vi "基本运动参考例程 - Copy.vi"() -> ()   [LabVIEW 2020]
uses:
  VIs/gts.lvlib
panel:
  in  "pPrm 3":cluster{"acc":dbl, "dec":dbl, "smooth":dbl}={"acc"=1.0, "dec"=1.0, "smooth"=0.0}
  in  "vel 2":dbl=30.0
  in  "Jog运动":bool
  in  "pos":i32=20000
  in  "vel":dbl=30.0
  in  "pPrm":T1={"acc"=1.0, "dec"=1.0, "velStart"=0.0, "smoothTime"=20}
  in  "点位运动":bool
  in  "数据路径":path
  in  "pCrdPrm":T2={"dimension"=2, "profile[0]"=1, "profile[1]"=2, "profile[2]"=0, "profile[3]"=0, "profile[4]"=0, "profile[5]"=0, "profile[6]"=0, "profile[7]"=0, "@dummy control@"=0, "@dummy control@"=0, "@dummy control@"=0, "@dummy control@"=0, "@dummy control@"=0, "@dummy control@"=0, "synVelMax"=500.0, "synAccMax"=1.0, "evenTime"=10, "setOriginFlag"=0, "originPos[0]"=0, "originPos[1]"=0, "originPos[2]"=0, "originPos[3]"=0, "originPos[4]"=0, "originPos[5]"=0, "originPos[6]"=0, "originPos[7]"=0}
  in  "前瞻":bool
  in  "插补运动":bool
  in  "pLookAheadBuf":T3(array[cluster])
  out "pStatus out":i16
  in  "轴号":T4(ring)=enum."1"
  in  "一维线性输出":bool
  in  "类型":u16(ring) items=["脉冲", "电平"]
  in  "单次输出":bool
  out "闭环返回值":i16[](array[numeric])
  in  "闭环PID参数":T5={"kp"=2.0, "ki"=0.0, "kd"=0.0, "kvff"=0.0, "kaff"=0.0, "integralLimit"=0, "derivativeLimit"=0, "limit"=32767}
  in  "闭环控制":bool
  out "updatemotion return":i16
  in  "更新运动":bool
  out "0号模块DI0输入":u16
  out "ExIoLoad return":i16
  out "openEXIO return":i16
  in  "扩展IO模块":bool
  out "2Dclear return":i16
  out "zero return":i16
  in  "清零":bool
  out "CrdStart return":i16
  out "二维输出次数":i32
  out "一维输出次数":i32[](array[numeric])
  out "1Dstatus return":i16
  in  "查询位置比较状态":bool
  out "2Dsetpara return":i16
  in  "二维位置比较参数设置":T6={"encx"=1, "ency"=2, "source"=1, "outputType"=0, "startLevel"=0, "time"=30, "maxerr"=100, "threshold"=0}
  out "se2Dcompare return":i16
  out "2Ddata return":i16
  in  "二维位置数组":cluster{"px":i32, "py":i32}[](array[cluster])=[{"px"=10000, "py"=10000}, {"px"=20000, "py"=20000}, {"px"=30000, "py"=30000}]
  out "1Dcompare return":i16
  in  "一维位置数组":dbl[](array[numeric])=[10000.0, 20000.0, 30000.0]
  out "crddata return":i16
  out "Lnxy return":i16
  out "setCrd return":i16
  out "lookahead":i16
  in  "二维位置比较":bool
  in  "一维位置比较":bool
  out "实际速度":dbl[](array[numeric])
  out "getenc return":i16
  out "实际位置":dbl[](array[numeric])
  out "encvel return":i16
  out "规划位置":dbl[](array[numeric])
  out "prfpos return":i16
  out "规划速度":dbl[](array[numeric])
  out "prfvel return":i16
  out "homezero return":i16
  out "gethomests return":i16
  out "pHomeStatus out":T7
  out "gohome return":i16
  out "get home prm return":i16
  in  "pHomePrm":T8={"mode"=20, "moveDir"=1, "indexDir"=1, "edge"=0, "triggerIndex"=-1, "pad1[0]"=0, "pad1[1]"=0, "pad1[2]"=0, "velHigh"=10.0, "velLow"=3.0, "acc"=0.1, "dec"=0.1, "smoothTime"=20, "pad2[0]"=0, "pad2[1]"=0, "pad2[2]"=0, "homeOffset"=1000, "searchHomeDistance"=0, "searchIndexDistance"=0, "escapeStep"=0, "pad3[0]"=0, "pad3[1]"=0}
  out "JogStop return":i16
  out "Update return":i16
  out "setVel return":i16
  out "setPrm return":i16
  out "getPrm return":i16
  out "PrfJog return":i16
  in  "回原点":bool
  out "reset return":i16
  out "Axisoff return":i16
  out "stopreturn":i16
  out "updatereturn":i16
  out "pos return":i16
  out "vel return":i16
  out "set prmreturn":i16
  out "get prm return":i16
  out "set trap return":i16
  out "Axison return":i16
  out "clrsts return":i16
  out "config return":i16
  in  "路径":path=path "D:/王淼清/控制卡常用功能例程(Labview)/GTS800.cfg"
  out "open return":i16
  in  "关伺服":bool
  in  "停止":bool
  in  "开伺服":bool
  in  "开卡":bool
  # "查询位置比较状态"
  # "插补运动参数"
  # "操作步骤：\n①按开卡键，打开卡和复位；\n②按开伺服键，1轴使能；\n③按点位键，1轴运动；\n注意事项：\n①按键时，时间不能太短，稍微长按一会；\n③在按键前，先设置各参数；\n④需要停止时，按停止键。\n参数说明：\naxis：运动轴，范围为1-8；\nvel：当前轴的轴速；\npos：当前轴的规划位置；\npPrm：点位运动的参数设置，可参考编程手册；\nconfig：配置文件，具体参数设置参考编程手册；\n备注：\n本例程函数返回值都以显示控件表示，函数名称在\n显示控件上方，每个函数都对应有一个显示控件，\n重复调用函数，只对应一个显示控件；"
  # "位置速度显示"
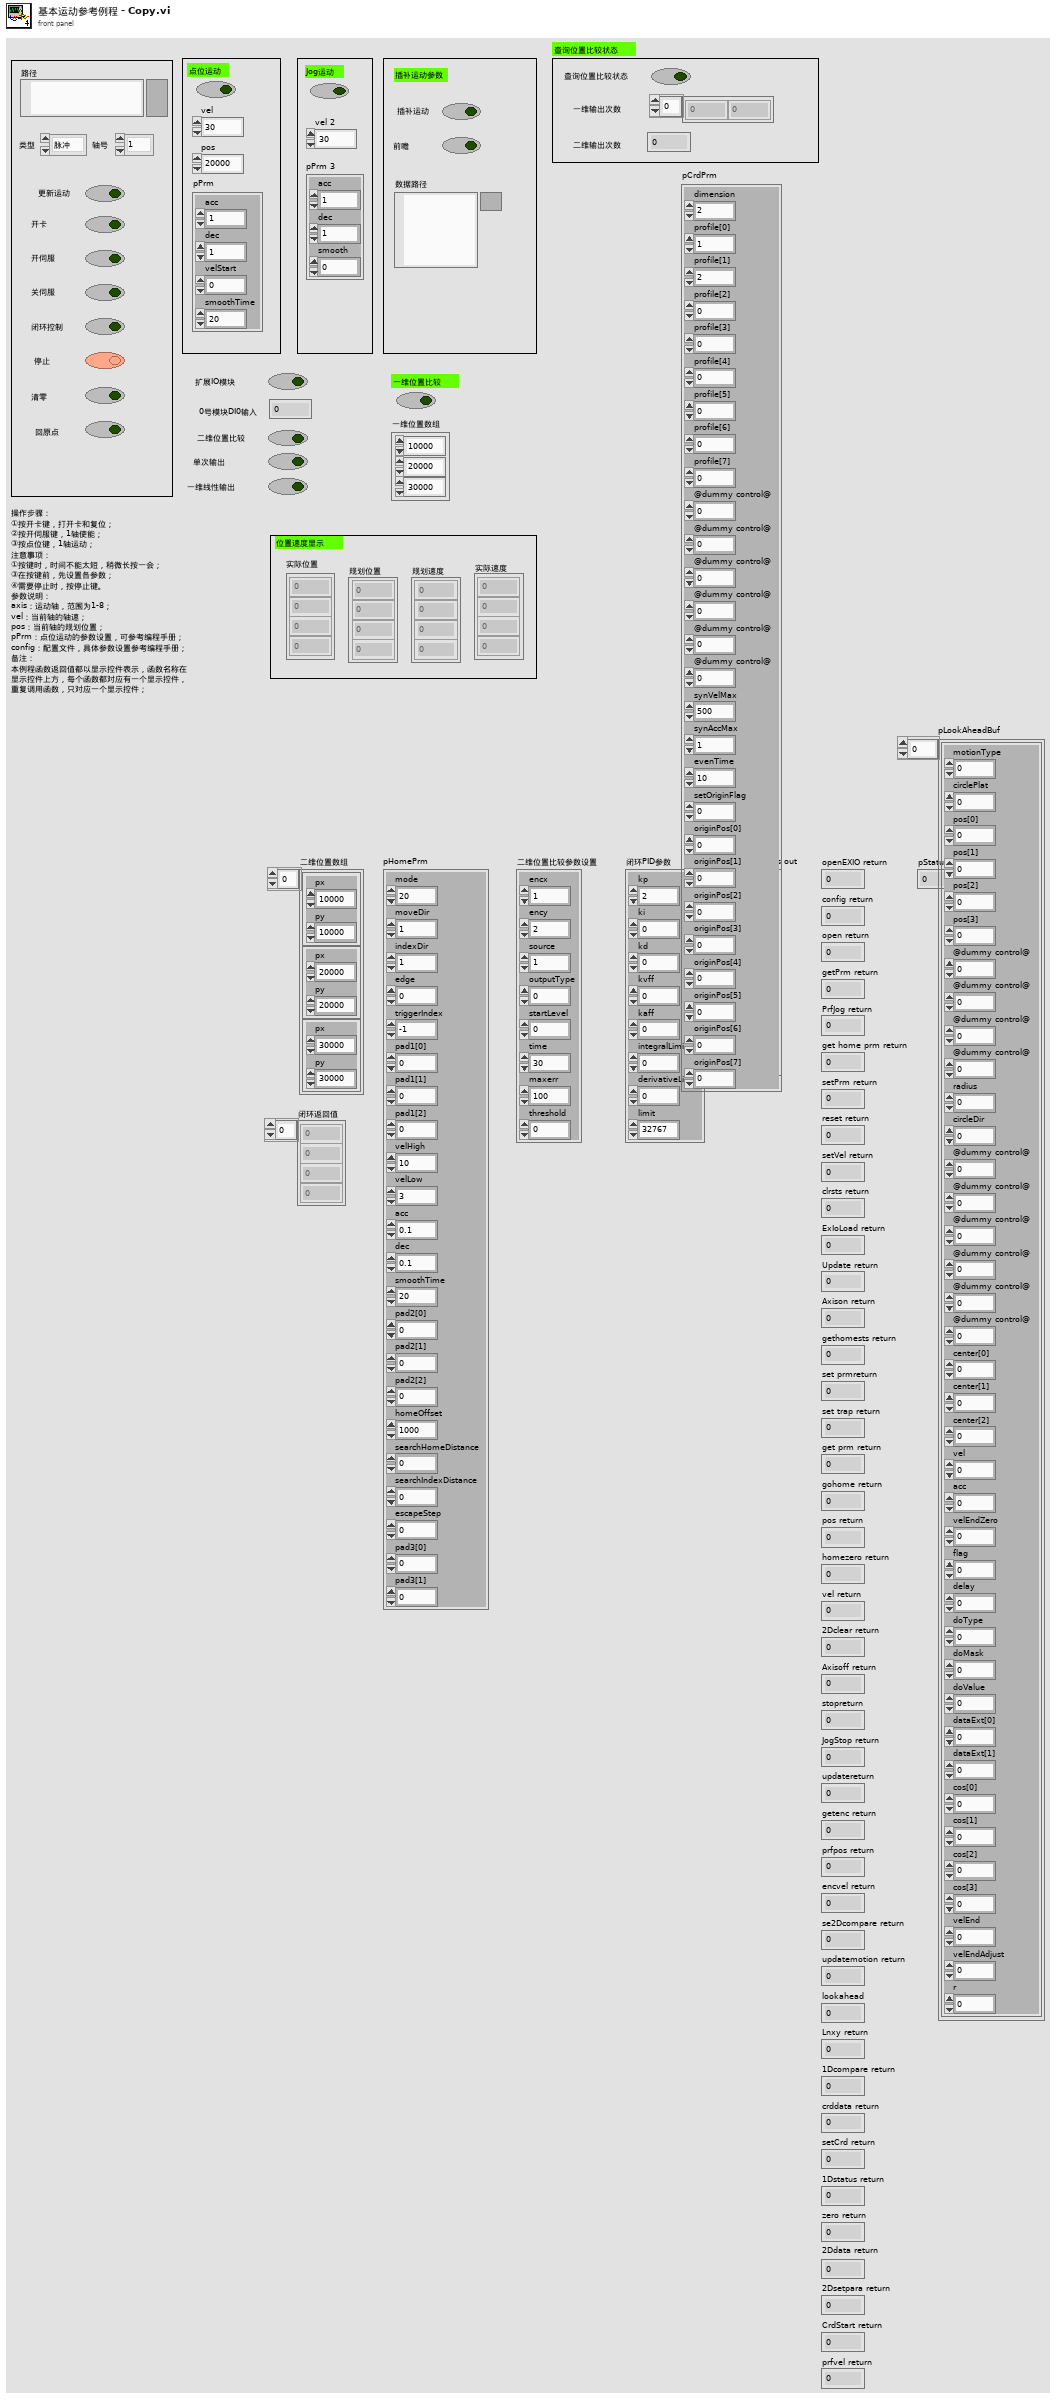
[diagram p1: front panel]
types:
  T1 = cluster{"acc":dbl, "dec":dbl, "velStart":dbl, "smoothTime":i16}
  T2 = cluster{"dimension":i16, "profile[0]":i16, "profile[1]":i16, "profile[2]":i16, "profile[3]":i16, "profile[4]":i16, "profile[5]":i16, "profile[6]":i16, "profile[7]":i16, "@dummy control@":i8, "@dummy control@":i8, "@dummy control@":i8, "@dummy control@":i8, "@dummy control@":i8, "@dummy control@":i8, "synVelMax":dbl, "synAccMax":dbl, "evenTime":i16, "setOriginFlag":i16, "originPos[0]":i32, "originPos[1]":i32, "originPos[2]":i32, "originPos[3]":i32, "originPos[4]":i32, "originPos[5]":i32, "originPos[6]":i32, "originPos[7]":i32}
  T3 = cluster{"motionType":i16, "circlePlat":i16, "pos[0]":i32, "pos[1]":i32, "pos[2]":i32, "pos[3]":i32, "@dummy control@":i8, "@dummy control@":i8, "@dummy control@":i8, "@dummy control@":i8, "radius":dbl, "circleDir":i16, "@dummy control@":i8, "@dummy control@":i8, "@dummy control@":i8, "@dummy control@":i8, "@dummy control@":i8, "@dummy control@":i8, "center[0]":dbl, "center[1]":dbl, "center[2]":dbl, "vel":dbl, "acc":dbl, "velEndZero":i16, "flag":i16, "delay":u16, "doType":i16, "doMask":u16, "doValue":u16, "dataExt[0]":u16, "dataExt[1]":u16, "cos[0]":dbl, "cos[1]":dbl, "cos[2]":dbl, "cos[3]":dbl, "velEnd":dbl, "velEndAdjust":dbl, "r":dbl}[]
  T4 = enum16{"none", "1", "2", "3", "4", "5", "6", "7", "8"}
  T5 = cluster{"kp":dbl, "ki":dbl, "kd":dbl, "kvff":dbl, "kaff":dbl, "integralLimit":i32, "derivativeLimit":i32, "limit":i16}
  T6 = cluster{"encx":i16, "ency":i16, "source":i16, "outputType":i16, "startLevel":i16, "time":i16, "maxerr":i16, "threshold":i16}
  T7 = cluster{"run":i16, "stage":i16, "error":i16, "pad1":i16, "capturePos":i32, "targetPos":i32}
  T8 = cluster{"mode":i16, "moveDir":i16, "indexDir":i16, "edge":i16, "triggerIndex":i16, "pad1[0]":i16, "pad1[1]":i16, "pad1[2]":i16, "velHigh":dbl, "velLow":dbl, "acc":dbl, "dec":dbl, "smoothTime":i16, "pad2[0]":i16, "pad2[1]":i16, "pad2[2]":i16, "homeOffset":i32, "searchHomeDistance":i32, "searchIndexDistance":i32, "escapeStep":i32, "pad3[0]":i32, "pad3[1]":i32}
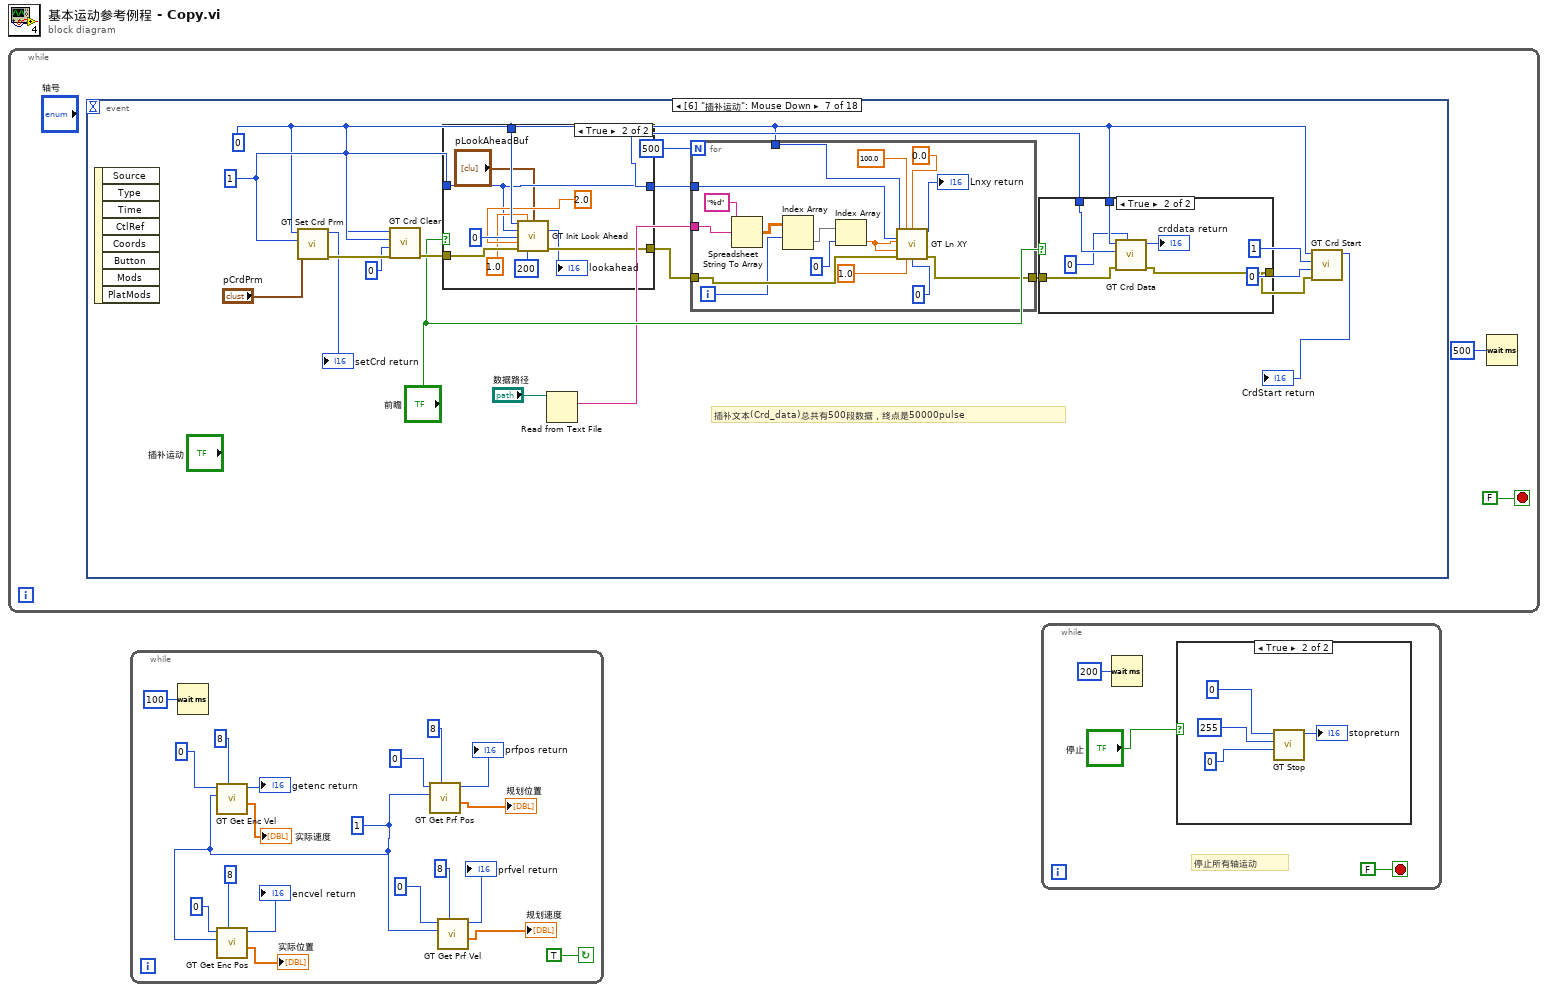
[diagram p0: block diagram]
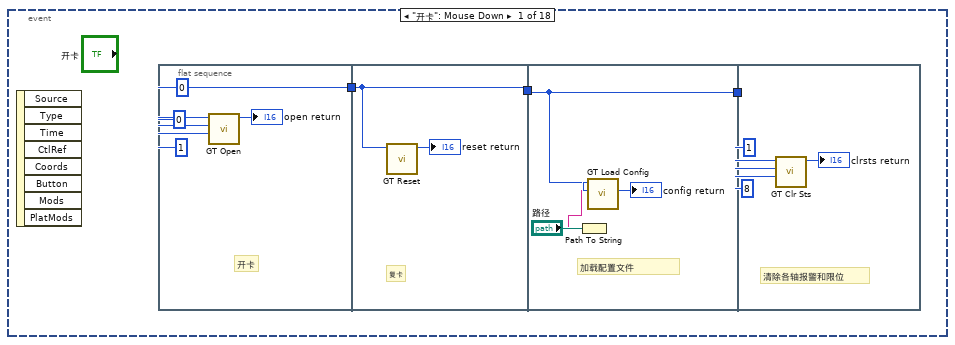
[diagram p3: hidden frame]
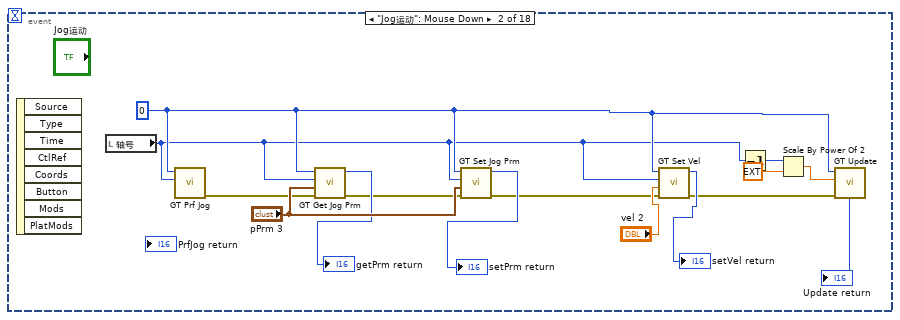
[diagram p4: hidden frame]
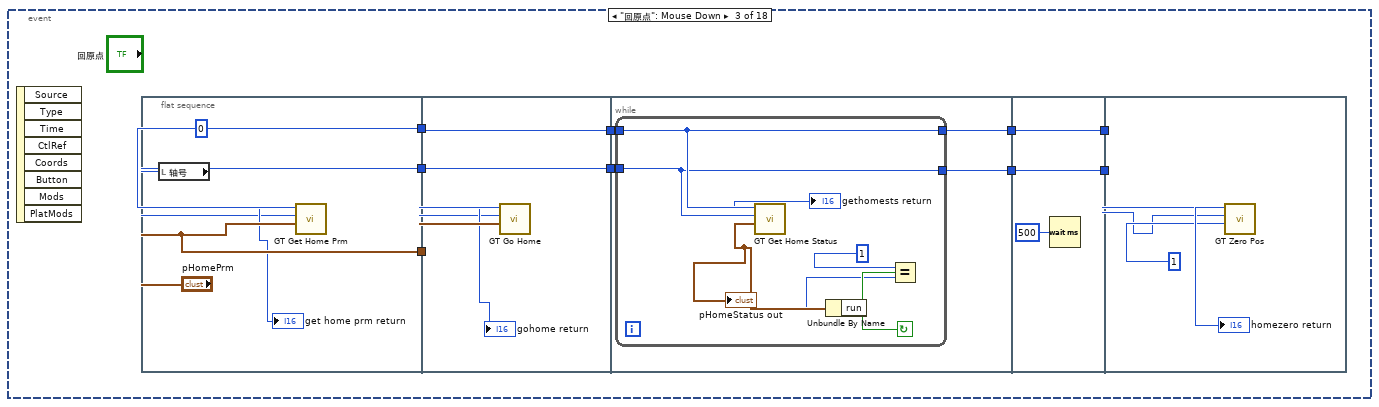
[diagram p5: hidden frame]
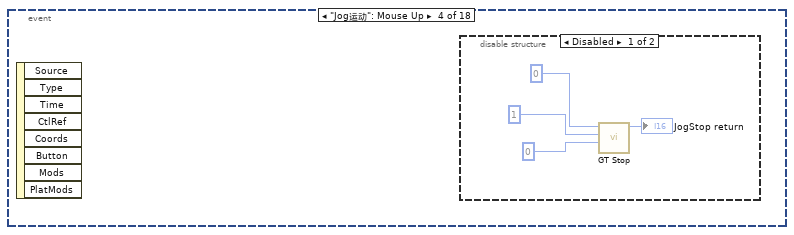
[diagram p6: hidden frame]
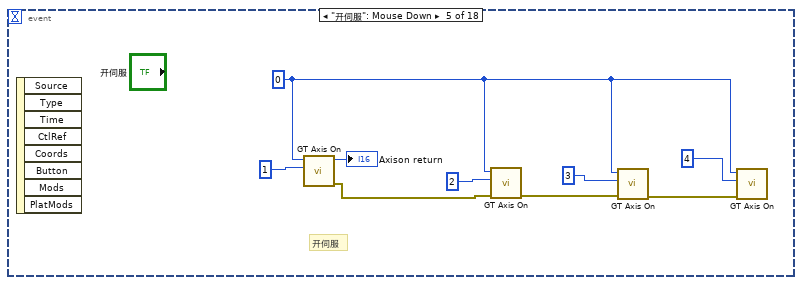
[diagram p8: hidden frame]
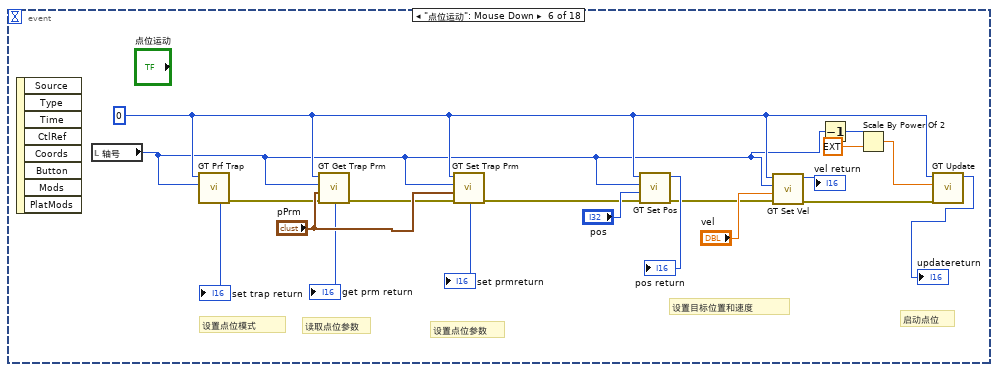
[diagram p9: hidden frame]
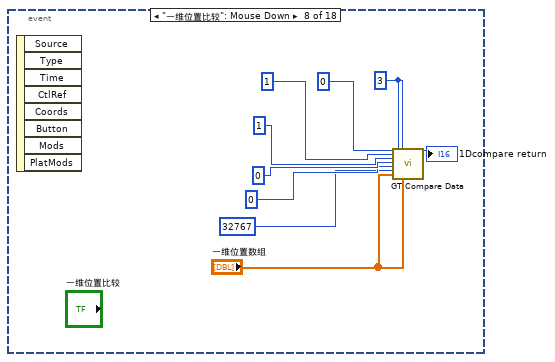
[diagram p12: hidden frame]
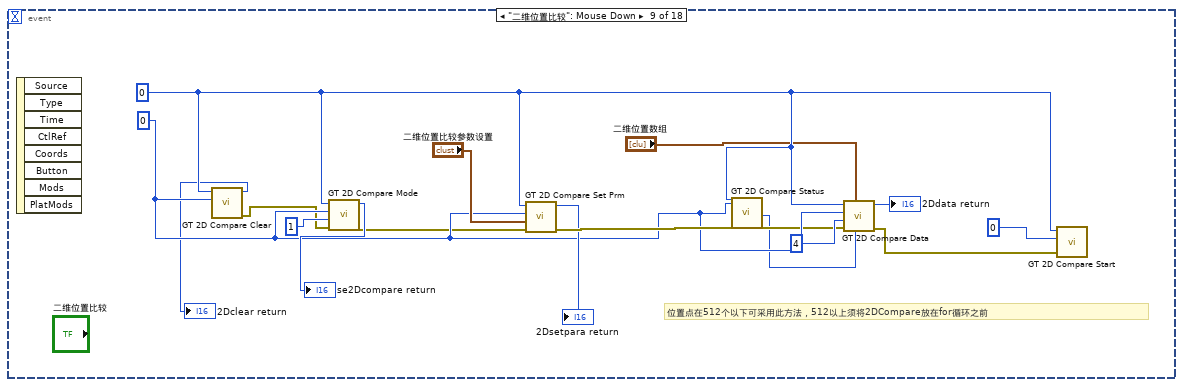
[diagram p13: hidden frame]
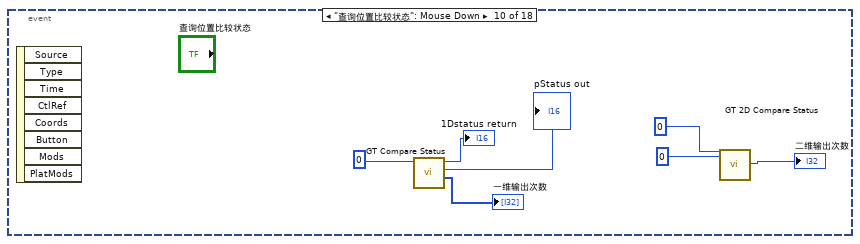
[diagram p14: hidden frame]
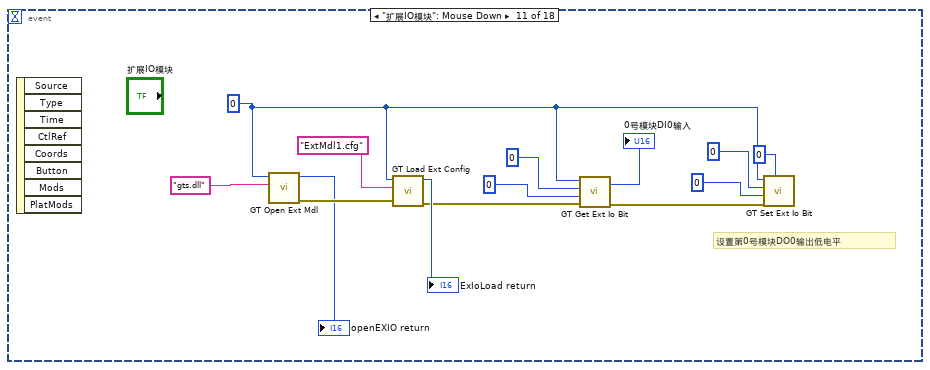
[diagram p15: hidden frame]
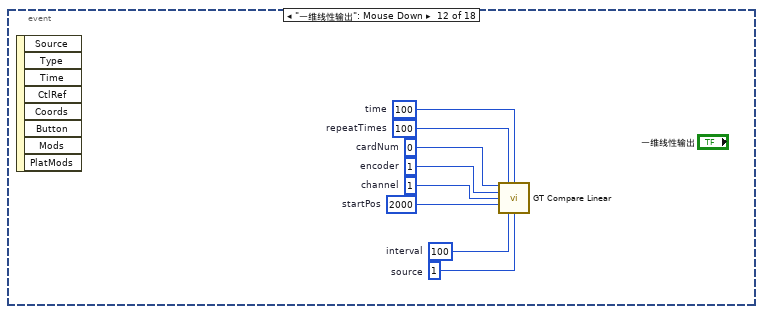
[diagram p16: hidden frame]
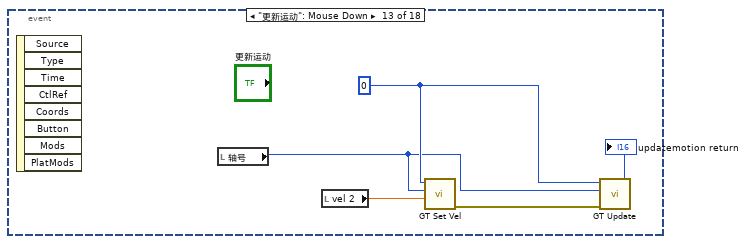
[diagram p17: hidden frame]
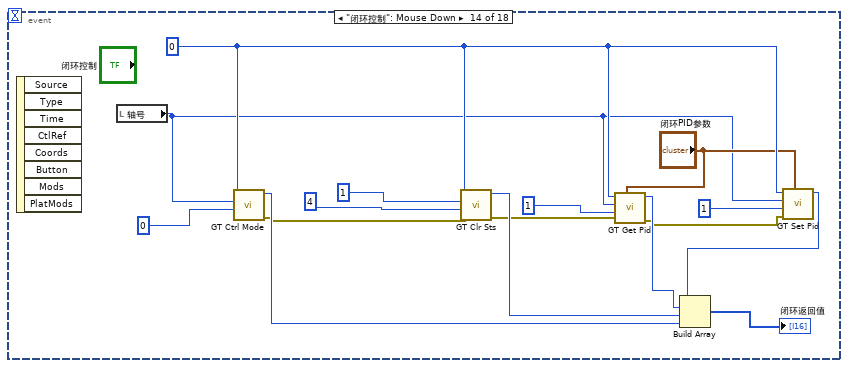
[diagram p18: hidden frame]
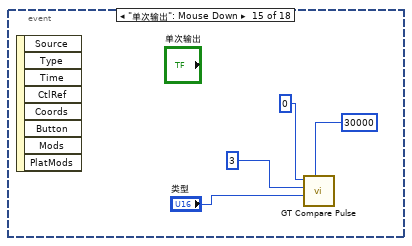
[diagram p19: hidden frame]
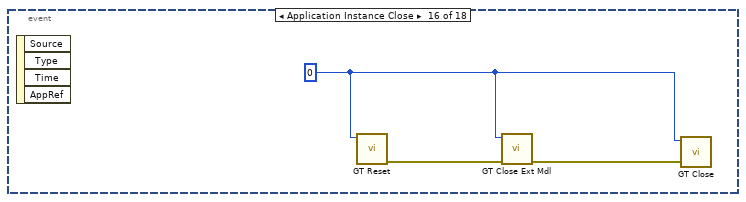
[diagram p20: hidden frame]
diagram:
  n1 = while {
    stop <- FALSE stop-if-true
    n2 = event shown="[6] \"插补运动\": Mouse Down" {
      selector: _ -> [_ _ _ _ _ _ _ _ _ _ _ _ _ _ _ _ _ _]
      dyn-events: _ -> [_ _ _ _ _ _ _ _ _ _ _ _ _ _ _ _ _ _]
      timeout: _ -> [_ _ _ _ _ _ _ _ _ _ _ _ _ _ _ _ _ _]
      event "开卡": Mouse Down {
        n3 = event-data() -> ()  [unwired: 1 in, 8 out]
        n4 = flat-sequence {
          tunnel: [w8] -> w5
          tunnel: w5 -> [w10]
          tunnel: [w10] -> w4
          tunnel: w4 -> [w12]
          tunnel: [w12] -> w3
          tunnel: w3 -> [w18]
          frame #0 {
            w8 = i16 0 ("channel")
            # "开卡"
            n5 = call "GT Open.vi"("param"=i16 1, "channel"=i16 0, "cardNum"=w8) -> ("function return"=→"open return":i16)  [unwired: 7 in, 1 out]
          }
          frame #1 {
            # "复卡"
            n6 = call "GT Reset.vi"("cardNum"=w10) -> ("function return"=→"reset return":i16)  [unwired: 9 in, 1 out]
          }
          frame #2 {
            # "加载配置文件"
            n7 = Path To String(path="路径") -> (string=w13:string)
            n8 = call "GT Load Config.vi"("pFile"=w13, "cardNum"=w12) -> ("function return"=→"config return":i16)  [unwired: 7 in, 2 out]
          }
          frame #3 {
            # "清除各轴报警和限位"
            n9 = call "GT Clr Sts.vi"("count"=i16 8, "axis"=i16 1, "cardNum"=w18) -> ("function return"=→"clrsts return":i16)  [unwired: 7 in, 1 out]
          }
        }
      }
      event "Jog运动": Mouse Down {
        w34 = i16 0 ("cardNum")
        n10 = event-data() -> ()  [unwired: 1 in, 8 out]
        n11 = local read "轴号"() -> (w21:T4)
        n12 = call "GT Prf Jog.vi"("profile"=w21, "cardNum"=w34) -> ("error out"=w32:errorcluster)  [unwired: 8 in, 1 out]
        n13 = call "GT Get Jog Prm.vi"("error in (no error)"=w32, "pPrm"="pPrm 3", "profile"=w21, "cardNum"=w34) -> ("error out"=w26:errorcluster, "function return"=→"getPrm return":i16)  [unwired: 5 in, 1 out]
        n14 = call "GT Set Jog Prm.vi"("error in (no error)"=w26, "pPrm"="pPrm 3", "profile"=w21, "cardNum"=w34) -> ("error out"=w25:errorcluster, "function return"=→"setPrm return":i16)  [unwired: 5 in, 1 out]
        n15 = call "GT Set Vel.vi"("error in (no error)"=w25, "vel"="vel 2", "profile"=w21, "cardNum"=w34) -> ("error out"=w24:errorcluster, "function return"=→"setVel return":i16)  [unwired: 6 in]
        n16 = Decrement(x=w21) -> (x-1=w23:T4)
        n17 = Scale By Power Of 2(n=w23, x=ext 1.0) -> (x*2^n=w20:ext)
        n18 = call "GT Update.vi"("error in (no error)"=w24, "mask"=w20, "cardNum"=w34) -> ("function return"=→"Update return":i16)  [unwired: 7 in, 1 out]
      }
      event "回原点": Mouse Down {
        n19 = event-data() -> ()  [unwired: 1 in, 8 out]
        n20 = flat-sequence {
          tunnel: [w47] -> w43
          tunnel: ["pHomePrm"] -> w41
          tunnel: [w44] -> w38
          tunnel: w43 -> [w51]
          tunnel: [w51] -> w42
          tunnel: w41 -> [w50]
          tunnel: w38 -> [w48]
          tunnel: [w48] -> w37
          tunnel: w42 -> [w55]
          tunnel: [w54] -> w40
          tunnel: w37 -> [w53]
          tunnel: [w52] -> w35
          tunnel: w40 -> [w65]
          tunnel: [w65] -> w39
          tunnel: [w63] -> w36
          tunnel: w35 -> [w63]
          tunnel: w39 -> [w67]
          tunnel: w36 -> [w66]
          frame #0 {
            w47 = i16 0 ("cardNum")
            n21 = local read "轴号"() -> (w44:T4)
            n22 = call "GT Get Home Prm.vi"("pHomePrm"="pHomePrm", "axis"=w44, "cardNum"=w47) -> ("function return"=→"get home prm return":i16)  [unwired: 6 in, 2 out]
          }
          frame #1 {
            n23 = call "GT Go Home.vi"("pHomePrm"=w50, "axis"=w48, "cardNum"=w51) -> ("function return"=→"gohome return":i16)  [unwired: 6 in, 2 out]
          }
          frame #2 {
            n24 = while {
              tunnel: w55 -> [w60]
              tunnel: [w60] -> w54
              tunnel: w53 -> [w56]
              tunnel: [w56] -> w52
              stop <- w61 continue-if-true
              n25 = call "GT Get Home Status.vi"("axis"=w56, "cardNum"=w60) -> ("pHomeStatus out"=w58:T7, "function return"=→"gethomests return":i16)  [unwired: 7 in, 1 out]
              "pHomeStatus out" <- w58
              n26 = Unbundle By Name(w58) -> ("run"=w57:i16)
              n27 = Equal?(x=i16 1, y=w57) -> (x = y?=w61:bool)
            }
          }
          frame #3 {
            n28 = Wait (ms)(milliseconds to wait=u32 500 ("等待时间（毫秒）")) -> ()  [unwired: 1 out]
          }
          frame #4 {
            n29 = call "GT Zero Pos.vi"("count"=i16 1, "axis"=w66, "cardNum"=w67) -> ("function return"=→"homezero return":i16)  [unwired: 7 in, 1 out]
          }
        }
      }
      event "Jog运动": Mouse Up {
        n30 = event-data() -> ()  [unwired: 1 in, 8 out]
        n31 = disable-structure shown="Disabled" {
          frame Disabled {
            n32 = call "GT Stop.vi"("option"=0, "mask"=1 ("option"), "cardNum"=0 ("mask")) -> ("function return"=→"JogStop return":i16)  [unwired: 7 in, 1 out]
          }
          frame Enabled {
          }
        }
      }
      event "开伺服": Mouse Down {
        w78 = i16 0 ("axis")
        # "开伺服"
        n33 = event-data() -> ()  [unwired: 1 in, 8 out]
        n34 = call "GT Axis On.vi"("axis"=i16 1, "cardNum"=w78) -> ("error out"=w79:errorcluster, "function return"=→"Axison return":i16)  [unwired: 8 in]
        n35 = call "GT Axis On.vi"("error in (no error)"=w79, "axis"=i16 2, "cardNum"=w78) -> ("error out"=w75:errorcluster)  [unwired: 7 in, 1 out]
        n36 = call "GT Axis On.vi"("error in (no error)"=w75, "axis"=i16 3, "cardNum"=w78) -> ("error out"=w74:errorcluster)  [unwired: 7 in, 1 out]
        n37 = call "GT Axis On.vi"("error in (no error)"=w74, "axis"=i16 4, "cardNum"=w78) -> ()  [unwired: 7 in, 2 out]
      }
      event "点位运动": Mouse Down {
        w89 = i16 0 ("cardNum")
        # "启动点位"
        # "设置目标位置和速度"
        # "设置点位参数"
        # "读取点位参数"
        # "设置点位模式"
        n38 = event-data() -> ()  [unwired: 1 in, 8 out]
        n39 = local read "轴号"() -> (w85:T4)
        n40 = call "GT Prf Trap.vi"("profile"=w85, "cardNum"=w89) -> ("error out"=w92:errorcluster, "function return"=→"set trap return":i16)  [unwired: 8 in]
        n41 = call "GT Get Trap Prm.vi"("error in (no error)"=w92, "pPrm"="pPrm", "profile"=w85, "cardNum"=w89) -> ("error out"=w91:errorcluster, "function return"=→"get prm return":i16)  [unwired: 5 in, 1 out]
        n42 = call "GT Set Trap Prm.vi"("error in (no error)"=w91, "pPrm"="pPrm", "profile"=w85, "cardNum"=w89) -> ("error out"=w90:errorcluster, "function return"=→"set prmreturn":i16)  [unwired: 5 in, 1 out]
        n43 = call "GT Set Pos.vi"("error in (no error)"=w90, "pos"="pos", "profile"=w85, "cardNum"=w89) -> ("error out"=w88:errorcluster, "function return"=→"pos return":i16)  [unwired: 6 in]
        n44 = call "GT Set Vel.vi"("error in (no error)"=w88, "vel"="vel", "profile"=w85, "cardNum"=w89) -> ("error out"=w87:errorcluster, "function return"=→"vel return":i16)  [unwired: 6 in]
        n45 = Decrement(x=w85) -> (x-1=w86:T4)
        n46 = Scale By Power Of 2(n=w86, x=ext 1.0) -> (x*2^n=w83:ext)
        n47 = call "GT Update.vi"("error in (no error)"=w87, "mask"=w83, "cardNum"=w89) -> ("function return"=→"updatereturn":i16)  [unwired: 7 in, 1 out]
      }
      event "插补运动": Mouse Down {
        w114 = i16 1 ("crd")
        w109 = i16 0 ("cardNum")
        # "插补文本(Crd_data)总共有500段数据，终点是50000pulse"
        n48 = event-data() -> ()  [unwired: 1 in, 8 out]
        n49 = call "GT Set Crd Prm.vi"("pCrdPrm"="pCrdPrm", "crd"=w114, "cardNum"=w109) -> ("error out"=w119:errorcluster, "function return"=→"setCrd return":i16)  [unwired: 7 in]
        n50 = call "GT Crd Clear.vi"("error in (no error)"=w119, "fifo"=i16 0, "crd"=w114, "cardNum"=w109) -> ("error out"=w117:errorcluster)  [unwired: 6 in, 1 out]
        n51 = case shown="True" "前瞻" {
          tunnel: w117 -> [w144 w154]
          tunnel: [w144 w153] -> w113
          tunnel: w109 -> [_ w152]
          tunnel: w114 -> [w143 w147]
          tunnel: [w143 w147] -> w111
          frame False {
          }
          frame True {
            n52 = call "GT Init Look Ahead.vi"("cardNum"=w152, "accMax"=1.0, "pLookAheadBuf"="pLookAheadBuf", "crd"=w147, "fifo"=i16 0, "T"=2.0, "error in (no error)"=w154, "n"=i16 200) -> ("function return"=→"lookahead":i16, "error out"=w153:errorcluster)  [unwired: 5 in, 1 out]
          }
        }
        n53 = Read from Text File(file (use dialog)="数据路径") -> (text=w103:string)  [unwired: 3 in, 3 out]
        n54 = for {
          N: 500 -> [_]
          tunnel: w111 -> [w123]
          tunnel: w109 -> [w122]
          tunnel: w103 -> [w127]
          tunnel: w113 -> [w135]
          tunnel: [w134] -> w110
          i -> [w125]
          n55 = Spreadsheet String To Array(format string="%d" ("格式字符串"), spreadsheet string=w127) -> (array=w126:dbl[][])  [unwired: 2 in]
          n56 = Index Array(array=w126, index (row)=w125) -> (element=w124:dbl[])  [unwired: 1 in]
          n57 = Index Array(array=w124, index=0 ("索引")) -> (element=w120:dbl)
          n58 = call "GT Ln XY.vi"("cardNum"=w122, "synVel"=100.0, "velEnd"=0.0, "crd"=w123, "x"=w120, "y"=w120, "error in (no error)"=w135, "synAcc"=1.0, "fifo"=i16 0) -> ("function return"=→"Lnxy return":i16, "error out"=w134:errorcluster)  [unwired: 5 in]
        }
        n59 = case shown="True" "前瞻" {
          tunnel: w109 -> [_ w142]
          tunnel: w111 -> [_ w141]
          tunnel: w110 -> [w136 w138]
          tunnel: [w136 w137] -> w105
          frame False {
          }
          frame True {
            n60 = call "GT Crd Data.vi"("fifo"=i16 0, "error in (no error)"=w138, "crd"=w141, "cardNum"=w142) -> ("error out"=w137:errorcluster, "function return"=→"crddata return":i16)  [unwired: 5 in, 1 out]
          }
        }
        n61 = call "GT Crd Start.vi"("error in (no error)"=w105, "option"=i16 0, "mask"=i16 1, "cardNum"=w109) -> ("function return"=→"CrdStart return":i16)  [unwired: 6 in, 1 out]
      }
      event "一维位置比较": Mouse Down {
        w155 = i16 3 ("count1")
        n62 = event-data() -> ()  [unwired: 1 in, 8 out]
        n63 = call "GT Compare Data.vi"("cardNum"=i16 0 ("cardnumber"), "encoder"=i16 1, "source"=i16 1, "pulseType"=i16 0, "startLevel"=i16 0, "time"=i16 32767, "pBuf1"="一维位置数组", "count1"=w155, "count2"=w155, "pBuf2"="一维位置数组") -> ("function return"=→"1Dcompare return":i16)  [unwired: 15 in, 2 out]
      }
      event "二维位置比较": Mouse Down {
        w173 = i16 0 ("chn")
        w174 = i16 0 ("cardNum")
        # "位置点在512个以下可采用此方法，512以上须将2DCompare放在for循环之前"
        n64 = event-data() -> ()  [unwired: 1 in, 8 out]
        n65 = call "GT 2D Compare Clear.vi"("chn"=w173, "cardNum"=w174) -> ("error out"=w171:errorcluster, "function return"=→"2Dclear return":i16)  [unwired: 8 in]
        n66 = call "GT 2D Compare Mode.vi"("error in (no error)"=w171, "mode"=i16 1, "chn"=w173, "cardNum"=w174) -> ("error out"=w170:errorcluster, "function return"=→"se2Dcompare return":i16)  [unwired: 6 in]
        n67 = call "GT 2D Compare Set Prm.vi"("error in (no error)"=w170, "pPrm"="二维位置比较参数设置", "chn"=w173, "cardNum"=w174) -> ("error out"=w178:errorcluster, "function return"=→"2Dsetpara return":i16)  [unwired: 5 in, 1 out]
        n68 = call "GT 2D Compare Status.vi"("cardNum"=w174, "chn"=w173, "error in (no error)"=w178) -> ("pFifo out"=w165:i16, "error out"=w166:errorcluster)  [unwired: 18 in, 5 out]
        n69 = call "GT 2D Compare Data.vi"("fifo"=w165, "pBuf"="二维位置数组", "error in (no error)"=w166, "count"=i16 4, "chn"=w173, "cardNum"=w174) -> ("error out"=w176:errorcluster, "function return"=→"2Ddata return":i16)  [unwired: 3 in, 1 out]
        n70 = call "GT 2D Compare Start.vi"("error in (no error)"=w176, "chn"=i16 0, "cardNum"=w174) -> ()  [unwired: 7 in, 2 out]
      }
      event "查询位置比较状态": Mouse Down {
        n71 = event-data() -> ()  [unwired: 1 in, 8 out]
        n72 = call "GT Compare Status.vi"("cardNum"=i16 0) -> ("pCount out"=→"一维输出次数":i32[], "pStatus out"=→"pStatus out":i16, "function return"=→"1Dstatus return":i16)  [unwired: 7 in, 1 out]
        n73 = call "GT 2D Compare Status.vi"("cardNum"=i16 0, "chn"=i16 0) -> ("pCount out"=→"二维输出次数":i32)  [unwired: 19 in, 6 out]
      }
      event "扩展IO模块": Mouse Down {
        w194 = i16 0 ("cardNum")
        # "设置第0号模块DO0输出低电平"
        n74 = event-data() -> ()  [unwired: 1 in, 8 out]
        n75 = call "GT Open Ext Mdl.vi"("pDllName"="gts.dll", "cardNum"=w194) -> ("error out"=w201:errorcluster, "function return"=→"openEXIO return":i16)  [unwired: 7 in, 1 out]
        n76 = call "GT Load Ext Config.vi"("error in (no error)"=w201, "pFileName"="ExtMdl1.cfg", "cardNum"=w194) -> ("error out"=w196:errorcluster, "function return"=→"ExIoLoad return":i16)  [unwired: 6 in, 1 out]
        n77 = call "GT Get Ext Io Bit.vi"("error in (no error)"=w196, "index"=i16 0, "mdl"=i16 0, "cardNum"=w194) -> ("error out"=w195:errorcluster, "pValue out"=→"0号模块DI0输入":u16)  [unwired: 5 in, 1 out]
        n78 = call "GT Set Ext Io Bit.vi"("value"=u16 0, "error in (no error)"=w195, "index"=i16 0, "mdl"=i16 0, "cardNum"=w194) -> ()  [unwired: 5 in, 2 out]
      }
      event "一维线性输出": Mouse Down {
        w202 = i16 1  # source
        w203 = 100  # interval
        w204 = i16 100  # time
        w205 = 100  # repeatTimes
        w206 = 2000  # startPos
        w207 = i16 1  # channel
        w208 = i16 1  # encoder
        w209 = i16 0  # cardNum
        n79 = event-data() -> ()  [unwired: 1 in, 8 out]
        n80 = call "GT Compare Linear.vi"("cardNum"=w209, "repeatTimes"=w205, "time"=w204, "encoder"=w208, "channel"=w207, "startPos"=w206, "interval"=w203, "source"=w202) -> ()  [unwired: 6 in, 2 out]
      }
      event "更新运动": Mouse Down {
        w212 = i16 0 ("cardNum")
        n81 = event-data() -> ()  [unwired: 1 in, 8 out]
        n82 = local read "轴号"() -> (w210:T4)
        n83 = local read "vel 2"() -> (w211:dbl)
        n84 = call "GT Set Vel.vi"("vel"=w211, "profile"=w210, "cardNum"=w212) -> ("error out"=w213:errorcluster)  [unwired: 7 in, 1 out]
        n85 = call "GT Update.vi"("error in (no error)"=w213, "mask"=w210, "cardNum"=w212) -> ("function return"=→"updatemotion return":i16)  [unwired: 7 in, 1 out]
      }
      event "闭环控制": Mouse Down {
        w219 = i16 0 ("cardNum")
        n86 = event-data() -> ()  [unwired: 1 in, 8 out]
        n87 = local read "轴号"() -> (w215:T4)
        n88 = call "GT Ctrl Mode.vi"("mode"=i16 0, "axis"=w215, "cardNum"=w219) -> ("error out"=w217:errorcluster, "function return"=w226:i16)  [unwired: 7 in]
        n89 = call "GT Clr Sts.vi"("error in (no error)"=w217, "count"=i16 4, "axis"=i16 1, "cardNum"=w219) -> ("error out"=w222:errorcluster, "function return"=w225:i16)  [unwired: 6 in]
        n90 = call "GT Get Pid.vi"("pPid"="闭环PID参数", "error in (no error)"=w222, "index"=i16 1, "control"=w215, "cardNum"=w219) -> ("error out"=w216:errorcluster, "function return"=w220:i16)  [unwired: 4 in, 1 out]
        n91 = call "GT Set Pid.vi"("pPid"="闭环PID参数", "error in (no error)"=w216, "index"=i16 1, "control"=w215, "cardNum"=w219) -> ("function return"=w224:i16)  [unwired: 4 in, 2 out]
        n92 = Build Array(w224, w220, w225, w226) -> (→"闭环返回值":i16[])
      }
      event "单次输出": Mouse Down {
        n93 = event-data() -> ()  [unwired: 1 in, 8 out]
        n94 = call "GT Compare Pulse.vi"("time"=i16 30000, "outputType"="类型", "level"=i16 3, "cardNum"=i16 0) -> ()  [unwired: 6 in, 2 out]
      }
      event Application Instance Close {
        w237 = i16 0 ("cardNum")
        n95 = event-data() -> ()  [unwired: 1 in, 4 out]
        n96 = call "GT Reset.vi"("cardNum"=w237) -> ("error out"=w236:errorcluster)  [unwired: 9 in, 1 out]
        n97 = call "GT Close Ext Mdl.vi"("error in (no error)"=w236, "cardNum"=w237) -> ("error out"=w235:errorcluster)  [unwired: 8 in, 1 out]
        n98 = call "GT Close.vi"("error in (no error)"=w235, "cardNum"=w237) -> ()  [unwired: 8 in, 2 out]
      }
      event "关伺服": Mouse Down {
        w242 = i16 0 ("axis")
        # "关伺服"
        n99 = event-data() -> ()  [unwired: 1 in, 8 out]
        n100 = call "GT Axis Off.vi"("axis"=i16 1, "cardNum"=w242) -> ("error out"=w243:errorcluster, "function return"=→"Axisoff return":i16)  [unwired: 8 in]
        n101 = call "GT Axis Off.vi"("error in (no error)"=w243, "axis"=i16 2, "cardNum"=w242) -> ("error out"=w241:errorcluster)  [unwired: 7 in, 1 out]
        n102 = call "GT Axis Off.vi"("error in (no error)"=w241, "axis"=i16 3, "cardNum"=w242) -> ("error out"=w240:errorcluster)  [unwired: 7 in, 1 out]
        n103 = call "GT Axis Off.vi"("error in (no error)"=w240, "axis"=i16 4, "cardNum"=w242) -> ()  [unwired: 7 in, 2 out]
      }
      event "清零": Mouse Down {
        n104 = event-data() -> ()  [unwired: 1 in, 8 out]
        n105 = call "GT Zero Pos.vi"("count"=i16 8, "axis"=i16 1, "cardNum"=i16 0) -> ("function return"=→"zero return":i16)  [unwired: 7 in, 1 out]
      }
    }
    n106 = Wait (ms)(milliseconds to wait=u32 500 ("等待时间（毫秒）")) -> ()  [unwired: 1 out]
  }
  n107 = while {
    stop <- TRUE continue-if-true
    w251 = i16 1 ("profile")
    n108 = Wait (ms)(milliseconds to wait=u32 100 ("等待时间（毫秒）")) -> ()  [unwired: 1 out]
    n109 = call "GT Get Enc Vel.vi"("count"=i16 8, "encoder"=w251, "cardNum"=i16 0 ("encoder")) -> ("pValue out"=→"实际速度":dbl[], "function return"=→"getenc return":i16)  [unwired: 5 in, 2 out]
    n110 = call "GT Get Enc Pos.vi"("count"=i16 8, "encoder"=w251, "cardNum"=i16 0 ("encoder")) -> ("pValue out"=→"实际位置":dbl[], "function return"=→"encvel return":i16)  [unwired: 5 in, 2 out]
    n111 = call "GT Get Prf Pos.vi"("count"=i16 8, "profile"=w251, "cardNum"=i16 0 ("profile")) -> ("pValue out"=→"规划位置":dbl[], "function return"=→"prfpos return":i16)  [unwired: 5 in, 2 out]
    n112 = call "GT Get Prf Vel.vi"("count"=i16 8, "profile"=w251, "cardNum"=i16 0 ("profile")) -> ("pValue out"=→"规划速度":dbl[], "function return"=→"prfvel return":i16)  [unwired: 5 in, 2 out]
  }
  n113 = while {
    stop <- FALSE stop-if-true
    # "停止所有轴运动"
    n114 = Wait (ms)(milliseconds to wait=u32 200 ("等待时间（毫秒）")) -> ()  [unwired: 1 out]
    n115 = case shown="True" "停止" {
      frame False {
      }
      frame True {
        n116 = call "GT Stop.vi"("option"=0, "mask"=255, "cardNum"=0 ("mask")) -> ("function return"=→"stopreturn":i16)  [unwired: 7 in, 1 out]
      }
    }
  }
